vi "Check For Incoming Commands.vi"(8 "Error In":errorcluster, 11 "Process In":refnum<class "Process.lvclass">) -> (0 "Error Out":errorcluster, 2 "New Command(s)":bool, 3 "Process Out":refnum<class "Process.lvclass">)   [LabVIEW 2019, in "Process.lvclass"]
uses:
  Process.lvclass
  Accessors/Message Queue/Get Message Queue.vi
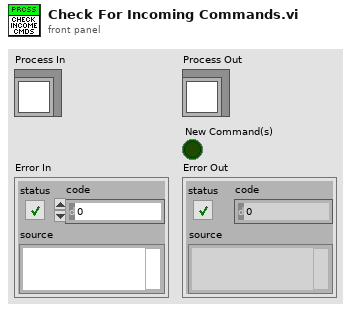
[diagram p1: front panel]
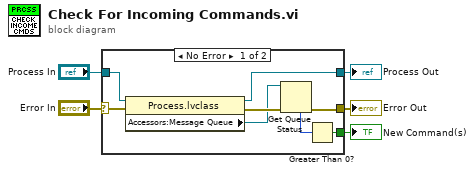
[diagram p0: block diagram]
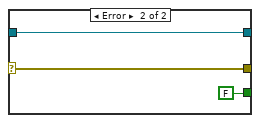
[diagram p2: hidden frame]
diagram:
  n1 = case shown="No Error" "Error In" {
    selector: "Error In" -> [w12 w16]
    tunnel: [w6 w16] -> w4
    tunnel: "Process In" -> [w13 w15]
    tunnel: [w9 w15] -> w2
    tunnel: [w7 FALSE] -> w1
    frame No Error {
      n2 = property class="Process.lvclass"(reference=w13, error in=w12) -> (reference out=w9:refnum<class "Process.lvclass">, error out=w11:errorcluster, "Accessors:Message Queue"=w10:refnum<queue>)
      n3 = Get Queue Status(queue=w10, error in (no error)=w11) -> (error out=w6:errorcluster, # elements in queue=w8:i32)  [unwired: 1 in, 6 out]
      n4 = Greater Than 0?(x=w8) -> (x > 0?=w7:bool)
    }
    frame Error {
    }
  }
  "Process Out" <- w2
  "Error Out" <- w4
  "New Command(s)" <- w1
